vi "Get Request Type.vi"(8 "error in (no error)":errorcluster, 11 "GetInputSettings in":refnum<class "GetInputSettings.lvclass">) -> (0 "error out":errorcluster, 2 "Request Type":string, 3 "GetInputSettings out":refnum<class "GetInputSettings.lvclass">)   [LabVIEW 2020, in "obs-websocket.lvlib" / "GetInputSettings.lvclass"]
uses:
  GetInputSettings.lvclass
  GetInputSettings.lvclass/GetInputSettings.ctl
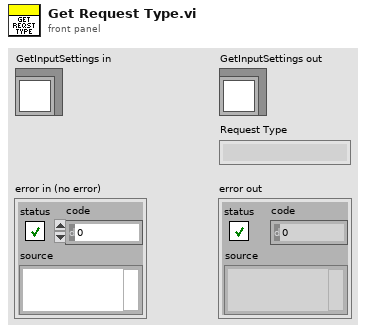
[diagram p1: front panel]
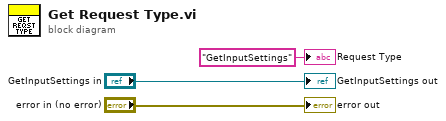
[diagram p0: block diagram]
diagram:
  "error out" <- "error in (no error)"
  "GetInputSettings out" <- "GetInputSettings in"
  "Request Type" <- "GetInputSettings" ("Request Type")
